vi "Get_Variable_Name.vi"(3 "Data":variant) -> (23 "Data Name(s)":string[](array[string]), 24 "Data Values(s)":string[](array[string]), 25 "Data Type(s)":string[](array[string]))   [LabVIEW 2011]
panel:
  out "xml string":string
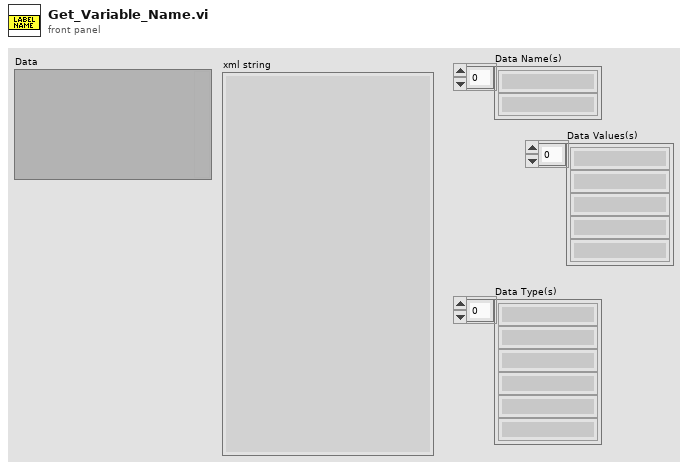
[diagram p1: front panel]
types:
  T1 = enum16{"XML Dimension Size", "XML Name", "XML Value"}
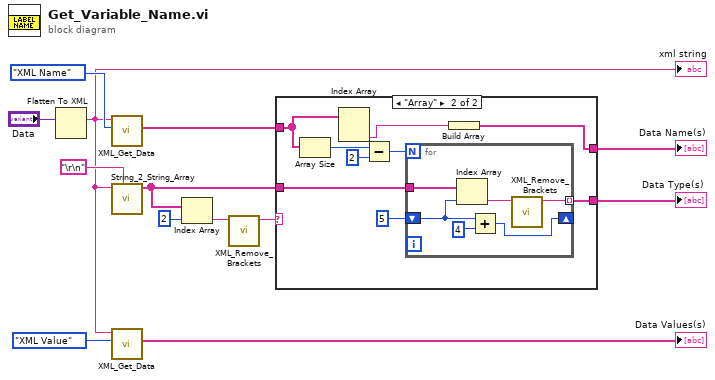
[diagram p0: block diagram]
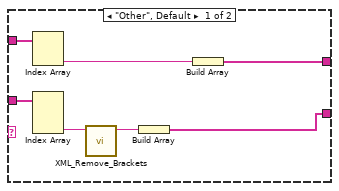
[diagram p2: hidden frame]
diagram:
  n1 = Flatten To XML(anything="Data") -> (xml string=w8:string)
  "xml string" <- w8
  n2 = call "XML_Get_Data.vi"("XML Data to Retrieve"=T1."XML Name", "XML String"=w8) -> ("XML Data"=w5:string[])  [unwired: 7 in, 2 out]
  n3 = call "String_2_String_Array.vi"("delimiter (;)"="\r\n", "String"=w8) -> ("String Array"=w2:string[])  [unwired: 9 in]
  n4 = call "XML_Get_Data.vi"("XML Data to Retrieve"=T1."XML Value", "XML String"=w8) -> ("XML Data"=→"Data Values(s)":string[])  [unwired: 7 in, 2 out]
  n5 = Index Array(array=w2, index=2) -> (element=w6:string)
  n6 = call "XML_Remove_Brackets.vi"("Input String"=w6) -> ("String without brackets"=w3:string)  [unwired: 10 in]
  n7 = case shown="\"Array\"" w3 {
    tunnel: w5 -> [w20 w23]
    tunnel: [w18 w21] -> w4
    tunnel: w2 -> [w17 w29]
    tunnel: [w14 w27] -> w1
    frame "Other", Default {
      n8 = Index Array(array=w20) -> (element #2=w19:string)  [unwired: 2 in, 1 out]
      n9 = Index Array(array=w17) -> (element #3=w16:string)  [unwired: 3 in, 2 out]
      n10 = call "XML_Remove_Brackets.vi"("Input String"=w16) -> ("String without brackets"=w15:string)  [unwired: 10 in]
      n11 = Build Array(w15) -> (w14:string[])
      n12 = Build Array(w19) -> (w18:string[])
    }
    frame "Array" {
      n13 = Array Size(array=w23) -> (size(s)=w25:i32)
      n14 = Index Array(array=w23) -> (element #2=w22:string)  [unwired: 2 in, 1 out]
      n15 = Subtract(x=w25, y=2 ("index")) -> (x-y=w26:i32)
      n16 = for {
        N: w26 -> [_]
        tunnel: w29 -> [w35]
        shift-right: [w32] -> _
        shift-left: 5 ("index") -> [w34]
        tunnel: [w30] -> w27 mode=indexing
        n17 = Index Array(array=w35, index=w34) -> (element=w31:string)
        n18 = Add(x=w34, y=4) -> (x+y=w32:i32)
        n19 = call "XML_Remove_Brackets.vi"("Input String"=w31) -> ("String without brackets"=w30:string)  [unwired: 10 in]
      }
      n20 = Build Array(w22) -> (w21:string[])
    }
  }
  "Data Name(s)" <- w4
  "Data Type(s)" <- w1
